vi "Base File Path.vi"() -> (3 "Paths Out":T1)   [LabVIEW 2021]
uses:
  File Paths.ctl
panel:
  in  "Paths":T1
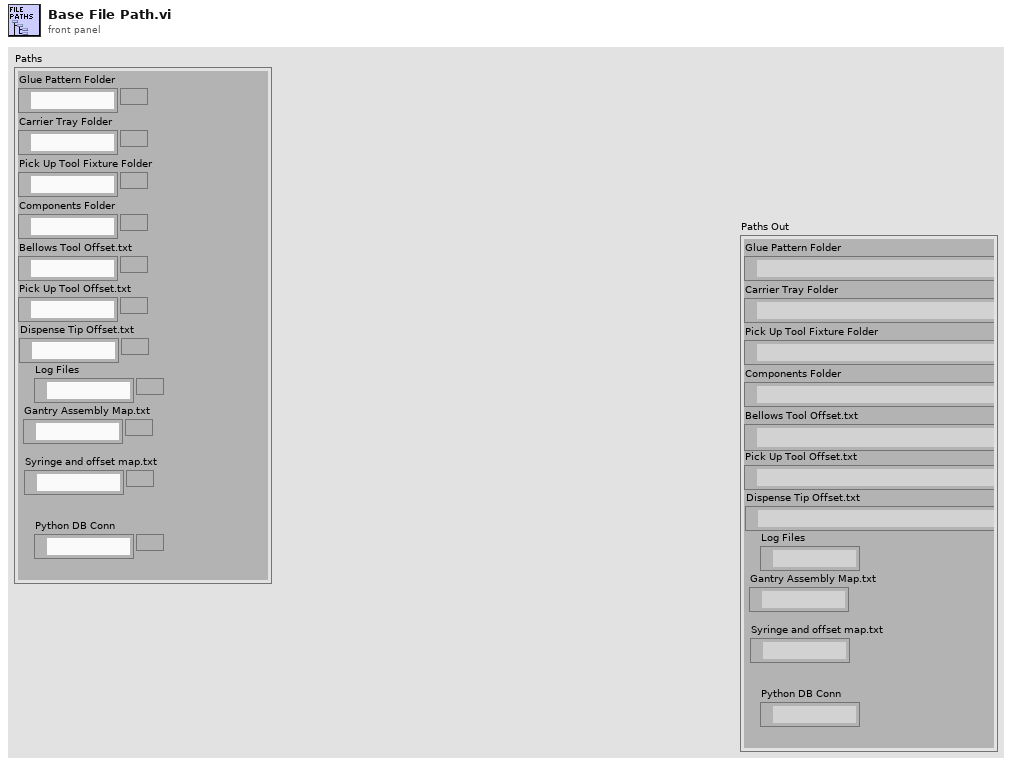
[diagram p1: front panel]
types:
  T1 = typedef "File Paths.ctl" = cluster{"Glue Pattern Folder":path, "Carrier Tray Folder":path, "Pick Up Tool Fixture Folder":path, "Components Folder":path, "Bellows Tool Offset.txt":path, "Pick Up Tool Offset.txt":path, "Dispense Tip Offset.txt":path, "Log Files":path, "Gantry Assembly Map.txt":path, "Syringe and offset map.txt":path, "Python DB Conn":path}
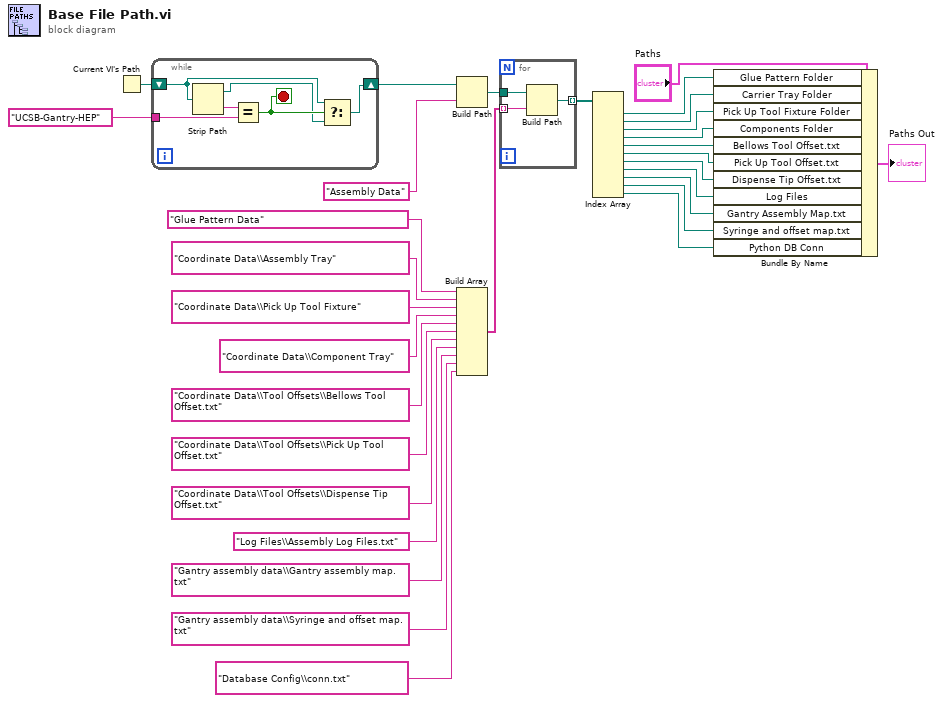
[diagram p0: block diagram]
diagram:
  n1 = Current VI's Path() -> (path=w31:path)
  n2 = while {
    shift-right: [w33] -> w27
    shift-left: w31 -> [w35]
    tunnel: "UCSB-Gantry-HEP" -> [w32]
    stop <- w36 stop-if-true
    n3 = Strip Path(path=w35) -> (stripped path=w34:path, name=w37:string)
    n4 = Equal?(x=w37, y=w32) -> (x = y?=w36:bool)
    n5 = Select(t=w35, s=w36, f=w34) -> (s? t:f=w33:path)
  }
  n6 = Build Path(base path=w27, name or relative path="Assembly Data") -> (appended path=w25:path)
  n7 = Build Array("Glue Pattern Data", "Coordinate Data\\Assembly Tray", "Coordinate Data\\Pick Up Tool Fixture", "Coordinate Data\\Component Tray" ("element"), "Coordinate Data\\Tool Offsets\\Bellows Tool Offset.txt", "Coordinate Data\\Tool Offsets\\Pick Up Tool Offset.txt", "Coordinate Data\\Tool Offsets\\Dispense Tip Offset.txt", "Log Files\\Assembly Log Files.txt", "Gantry assembly data\\Gantry assembly map.txt", "Gantry assembly data\\Syringe and offset map.txt", "Database Config\\conn.txt") -> (w17:string[])
  n8 = for {
    tunnel: w25 -> [w40]
    tunnel: [w39] -> w29 mode=indexing
    tunnel: w17 -> [w38] mode=indexing
    n9 = Build Path(base path=w40, name or relative path=w38) -> (appended path=w39:path)
  }
  n10 = Index Array(array=w29) -> (element #1=w16:path, element #2=w15:path, element #3=w14:path, element #4=w13:path, element #5=w12:path, element #6=w11:path, element #7=w10:path, element #8=w7:path, element #9=w4:path, element #10=w3:path, element #11=w2:path)  [unwired: 11 in]
  n11 = Bundle By Name(cluster="Paths", "Glue Pattern Folder"=w16, "Carrier Tray Folder"=w15, "Pick Up Tool Fixture Folder"=w14, "Components Folder"=w13, "Bellows Tool Offset.txt"=w12, "Pick Up Tool Offset.txt"=w11, "Dispense Tip Offset.txt"=w10, "Log Files"=w7, "Gantry Assembly Map.txt"=w4, "Syringe and offset map.txt"=w3, "Python DB Conn"=w2) -> (→"Paths Out":T1)
